vi "Errror on bit.vi"(8 "error in (no error)":errorcluster, 11 "ISO 14443 A DOWN in":refnum<class "ISO 14443 A DOWN.lvclass">) -> (0 "error out":errorcluster, 2 "Error on byte":dbl, 3 "ISO 14443 A DOWN out":refnum<class "ISO 14443 A DOWN.lvclass">)   [LabVIEW 2019, in "ISO 14443 A DOWN.lvclass"]
uses:
  ISO 14443 A DOWN.lvclass
  ISO 14443 A DOWN.lvclass/ISO 14443 A DOWN.ctl
  <userlib>/_OpenG.lib/array/array.llb/Filter 1D Array with Scalar (Boolean)__ogtk.vi
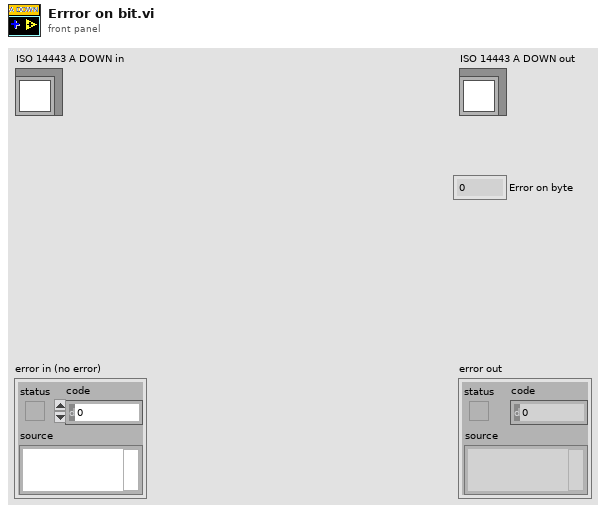
[diagram p1: front panel]
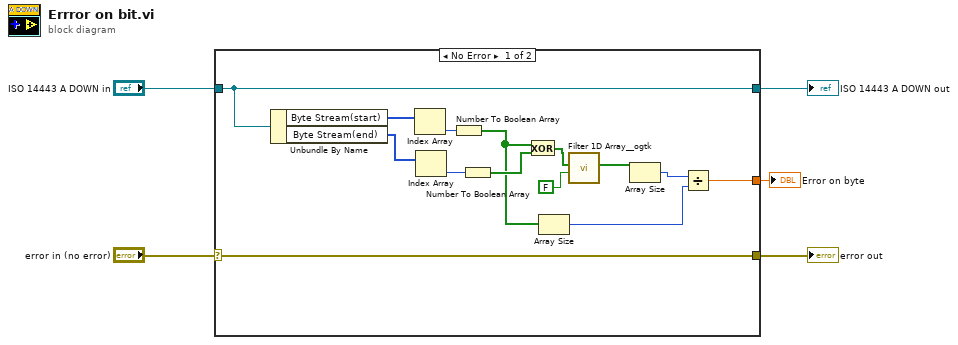
[diagram p0: block diagram]
diagram:
  n1 = case shown="No Error" "error in (no error)" {
    selector: "error in (no error)" -> [w19 w20]
    tunnel: "ISO 14443 A DOWN in" -> [w18 w21]
    tunnel: [w18 w21] -> w3
    tunnel: [w19 w20] -> w2
    tunnel: [w8 _] -> w1
    frame No Error {
      n2 = Unbundle By Name(w18) -> ("Byte Stream(start)"=w17:u8[], "Byte Stream(end)"=w16:u8[])
      n3 = Index Array(array=w17) -> (element=w7:u8)  [unwired: 1 in]
      n4 = Index Array(array=w16) -> (element=w15:u8)  [unwired: 1 in]
      n5 = Number To Boolean Array(number=w7) -> (Boolean array=w6:bool[])
      n6 = Number To Boolean Array(number=w15) -> (Boolean array=w14:bool[])
      n7 = Exclusive Or(1:w14, 2:w6) -> (0:w13:bool[])
      n8 = Array Size(array=w6) -> (size(s)=w9:i32)
      n9 = call-poly <userlib>:"Filter 1D Array__ogtk.vi"("items to filter"=FALSE, "array"=w13) -> ("filtered array"=w11:bool[])  [unwired: 4 in, 1 out]
      n10 = Array Size(array=w11) -> (size(s)=w10:i32)
      n11 = Divide(x=w10, y=w9) -> (x/y=w8:dbl)
    }
    frame Error {
    }
  }
  "error out" <- w2
  "ISO 14443 A DOWN out" <- w3
  "Error on byte" <- w1
